vi "data2image_4d.vi"(10 "image_4d":sgl[][][][](array[numeric])) -> (2 "image_1d":sgl[](array[numeric]))   [LabVIEW 2014]
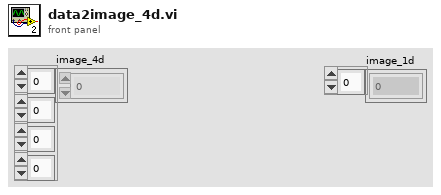
[diagram p1: front panel]
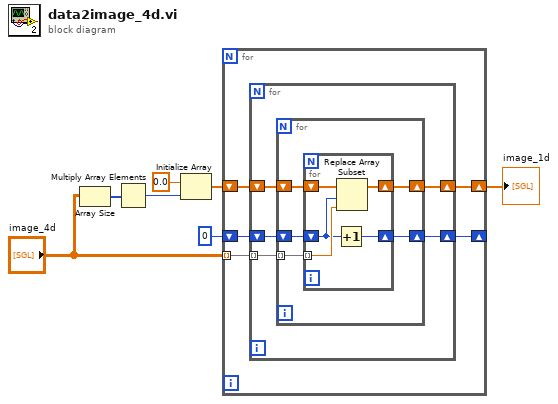
[diagram p0: block diagram]
diagram:
  n1 = Array Size(array="image_4d") -> (size(s)=w3:i32[])
  n2 = Multiply Array Elements(1:w3) -> (0:w4:i32)
  n3 = Initialize Array(sgl 0.0 ("element"), w4) -> (w6:sgl[])
  n4 = for {
    tunnel: "image_4d" -> [w12] mode=indexing
    shift-right: [w9] -> w1
    shift-left: w6 -> [w10]
    shift-right: [w8] -> _
    shift-left: 0 -> [w11]
    n5 = for {
      tunnel: w12 -> [w17] mode=indexing
      shift-right: [w16] -> w8
      shift-left: w11 -> [w15]
      shift-right: [w13] -> w9
      shift-left: w10 -> [w14]
      n6 = for {
        tunnel: w17 -> [w22] mode=indexing
        shift-right: [w21] -> w16
        shift-left: w15 -> [w20]
        shift-right: [w18] -> w13
        shift-left: w14 -> [w19]
        n7 = for {
          tunnel: w22 -> [w25] mode=indexing
          shift-right: [w27] -> w21
          shift-left: w20 -> [w24]
          shift-right: [w23] -> w18
          shift-left: w19 -> [w26]
          n8 = Increment(x=w24) -> (x+1=w27:i32)
          n9 = Replace Array Subset(array=w26, new element=w25, index=w24) -> (w23:sgl[])
        }
      }
    }
  }
  "image_1d" <- w1
